vi "Track_overlay_test.vi"() -> ()   [LabVIEW 2018]
uses:
  Tracker.lvlib
panel:
  out "Color":u32(colorbox)=16711680
  out "Image Display 2":T1(plugin-control)
  out "Image Display":T1(plugin-control)
  out "error out":errorcluster
  in  "error in (no error)":errorcluster
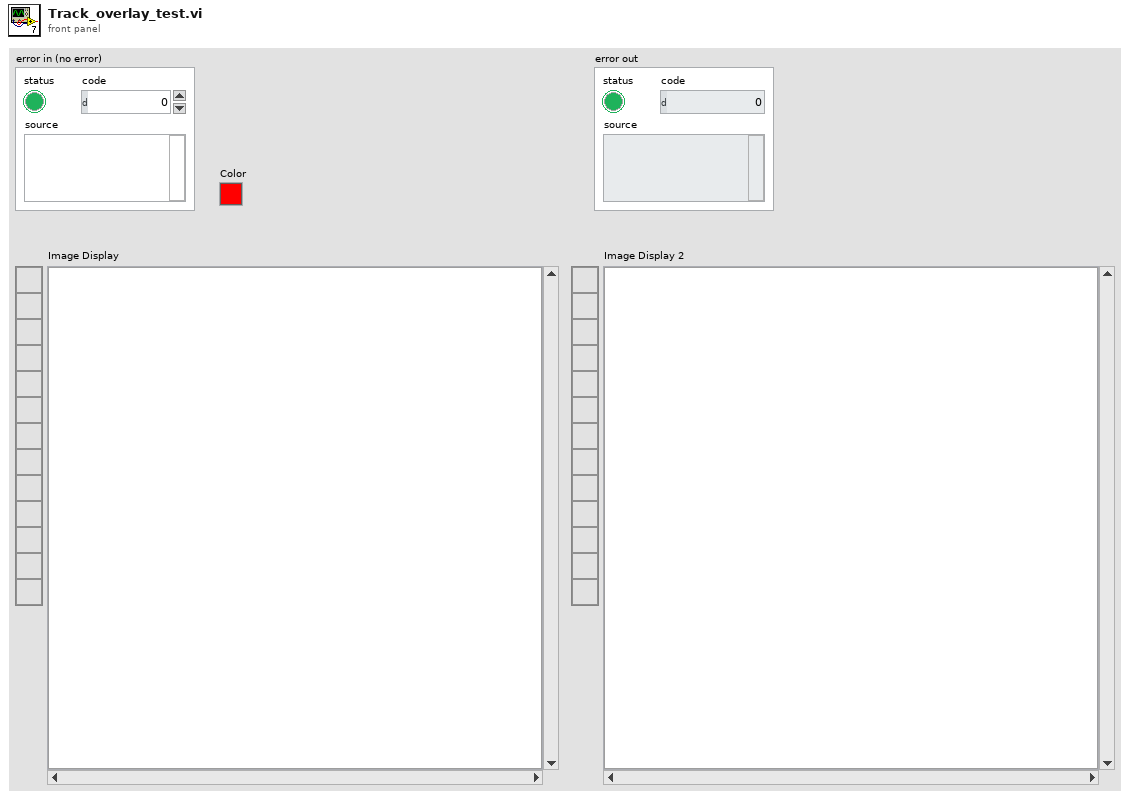
[diagram p1: front panel]
types:
  T1 = typedef "IMAQ Image.ctl" = refnum<image>
  T2 = cluster{"Left":i32, "Top":i32, "Right":i32, "Bottom":i32}
  T3 = typedef "Image Type" = u32
  T4 = cluster{"Numeric Control":dbl, "Numeric Control":dbl}[]
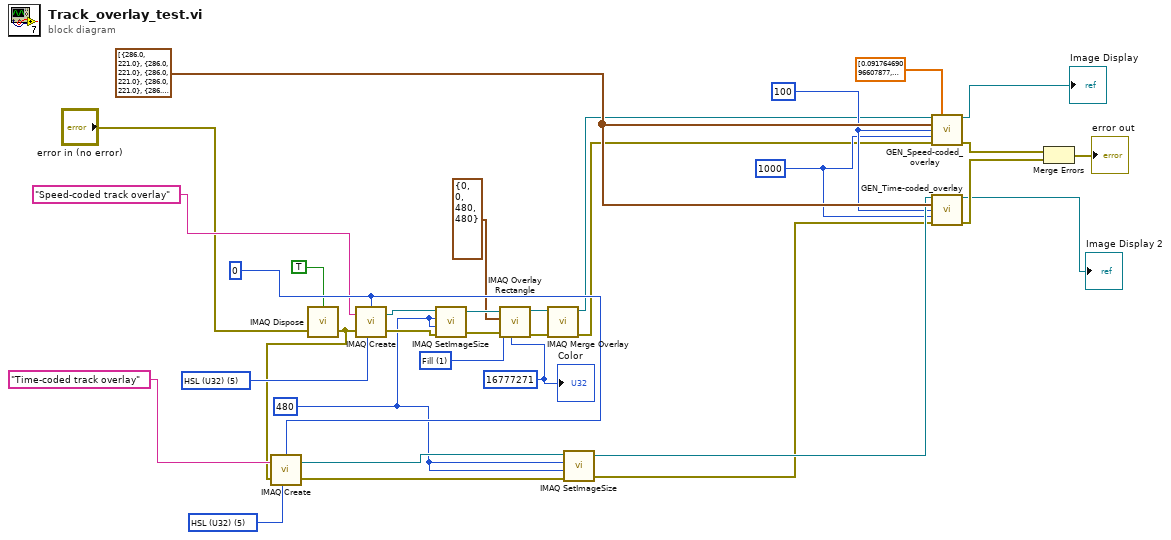
[diagram p0: block diagram]
diagram:
  w3 = u32 1 items=["Frame", "Fill", "Highlight"] ("Drawing Mode (Frame)")
  w5 = 16777271
  w21 = 0 ("Border Size")
  w23 = 1000 ("Samples full merge, every N")
  w24 = 100 ("Multiline grouping, samples")
  w18 = 480 ("X Resolution")
  w27 = T3 5 items=["Grayscale (U8)", "Grayscale (I16)", "Grayscale (SGL)", "Complex (CSG)", "RGB (U32)", "HSL (U32)", "RGB (U64)", "Grayscale (U16)"] ("Image Type")
  w20 = T3 5 items=["Grayscale (U8)", "Grayscale (I16)", "Grayscale (SGL)", "Complex (CSG)", "RGB (U32)", "HSL (U32)", "RGB (U64)", "Grayscale (U16)"] ("Image Type")
  w33 = T4 [{"Numeric Control"=286.0, "Numeric Control"=221.0}, {"Numeric Control"=286.0, "Numeric Control"=221.0}, {"Numeric Control"=286.0, "Numeric Control"=221.0}, {"Numeric Control"=286.0, "Numeric Control"=221.0}, {"Numeric Control"=286.0, "Numeric Control"=221.0}, {"Numeric Control"=286.0, "Numeric Control"=221.0}, {"Numeric Control"=286.0, "Numeric Control"=221.0}, {"Numeric Control"=286.0, "Numeric Control"=221.0}, {"Numeric Control"=286.0, "Numeric Control"=221.0}, {"Numeric Control"=285.0, "Numeric Control"=221.0}, {"Numeric Control"=285.0, "Numeric Control"=221.0}, {"Numeric Control"=285.0, "Numeric Control"=221.0}, {"Numeric Control"=285.0, "Numeric Control"=221.0}, {"Numeric Control"=285.0, "Numeric Control"=221.0}, {"Numeric Control"=285.0, "Numeric Control"=221.0}, {"Numeric Control"=285.0, "Numeric Control"=221.0}, {"Numeric Control"=285.0, "Numeric Control"=221.0}, {"Numeric Control"=285.0, "Numeric Control"=221.0}, {"Numeric Control"=285.0, "Numeric Control"=221.0}, {"Numeric Control"=285.0, "Numeric Control"=221.0}, {"Numeric Control"=285.0, "Numeric Control"=221.0}, {"Numeric Control"=285.0, "Numeric Control"=221.0}, {"Numeric Control"=285.0, "Numeric Control"=221.0}, {"Numeric Control"=285.0, "Numeric Control"=221.0}, {"Numeric Control"=285.0, "Numeric Control"=221.0}, {"Numeric Control"=285.0, "Numeric Control"=221.0}, {"Numeric Control"=286.0, "Numeric Control"=221.0}, {"Numeric Control"=286.0, "Numeric Control"=221.0}, {"Numeric Control"=285.0, "Numeric Control"=221.0}, {"Numeric Control"=286.0, "Numeric Control"=221.0}, {"Numeric Control"=286.0, "Numeric Control"=221.0}, {"Numeric Control"=286.0, "Numeric Control"=221.0}, {"Numeric Control"=285.0, "Numeric Control"=221.0}, {"Numeric Control"=286.0, "Numeric Control"=221.0}, {"Numeric Control"=286.0, "Numeric Control"=221.0}, {"Numeric Control"=286.0, "Numeric Control"=221.0}, {"Numeric Control"=286.0, "Numeric Control"=221.0}, {"Numeric Control"=286.0, "Numeric Control"=221.0}, {"Numeric Control"=286.0, "Numeric Control"=221.0}, {"Numeric Control"=286.0, "Numeric Control"=221.0}, {"Numeric Control"=286.0, "Numeric Control"=221.0}, {"Numeric Control"=286.0, "Numeric Control"=221.0}, {"Numeric Control"=286.0, "Numeric Control"=221.0}, {"Numeric Control"=286.0, "Numeric Control"=221.0}, {"Numeric Control"=286.0, "Numeric Control"=221.0}, {"Numeric Control"=286.0, "Numeric Control"=221.0}, {"Numeric Control"=285.0, "Numeric Control"=221.0}, {"Numeric Control"=285.0, "Numeric Control"=221.0}, {"Numeric Control"=285.0, "Numeric Control"=221.0}, {"Numeric Control"=285.0, "Numeric Control"=221.0}, {"Numeric Control"=285.0, "Numeric Control"=220.0}, {"Numeric Control"=285.0, "Numeric Control"=220.0}, {"Numeric Control"=285.0, "Numeric Control"=220.0}, {"Numeric Control"=285.0, "Numeric Control"=220.0}, {"Numeric Control"=285.0, "Numeric Control"=220.0}, {"Numeric Control"=285.0, "Numeric Control"=220.0}, {"Numeric Control"=285.0, "Numeric Control"=220.0}, {"Numeric Control"=285.0, "Numeric Control"=220.0}, {"Numeric Control"=285.0, "Numeric Control"=220.0}, {"Numeric Control"=285.0, "Numeric Control"=220.0}, {"Numeric Control"=285.0, "Numeric Control"=220.0}, {"Numeric Control"=285.0, "Numeric Control"=221.0}, {"Numeric Control"=285.0, "Numeric Control"=221.0}, {"Numeric Control"=285.0, "Numeric Control"=221.0}, {"Numeric Control"=285.0, "Numeric Control"=221.0}, {"Numeric Control"=285.0, "Numeric Control"=221.0}, {"Numeric Control"=285.0, "Numeric Control"=221.0}, {"Numeric Control"=285.0, "Numeric Control"=221.0}, {"Numeric Control"=285.0, "Numeric Control"=221.0}, {"Numeric Control"=285.0, "Numeric Control"=221.0}, {"Numeric Control"=285.0, "Numeric Control"=221.0}, {"Numeric Control"=286.0, "Numeric Control"=221.0}, {"Numeric Control"=286.0, "Numeric Control"=221.0}, {"Numeric Control"=286.0, "Numeric Control"=221.0}, {"Numeric Control"=286.0, "Numeric Control"=221.0}, {"Numeric Control"=286.0, "Numeric Control"=221.0}, {"Numeric Control"=286.0, "Numeric Control"=221.0}, {"Numeric Control"=286.0, "Numeric Control"=221.0}, {"Numeric Control"=286.0, "Numeric Control"=221.0}, {"Numeric Control"=286.0, "Numeric Control"=221.0}, {"Numeric Control"=286.0, "Numeric Control"=221.0}, {"Numeric Control"=286.0, "Numeric Control"=221.0}, {"Numeric Control"=286.0, "Numeric Control"=221.0}, {"Numeric Control"=286.0, "Numeric Control"=221.0}, {"Numeric Control"=286.0, "Numeric Control"=221.0}, {"Numeric Control"=286.0, "Numeric Control"=221.0}, {"Numeric Control"=286.0, "Numeric Control"=221.0}, {"Numeric Control"=286.0, "Numeric Control"=221.0}, {"Numeric Control"=286.0, "Numeric Control"=221.0}, {"Numeric Control"=286.0, "Numeric Control"=221.0}, {"Numeric Control"=286.0, "Numeric Control"=221.0}, {"Numeric Control"=286.0, "Numeric Control"=221.0}, {"Numeric Control"=286.0, "Numeric Control"=221.0}, {"Numeric Control"=286.0, "Numeric Control"=221.0}, {"Numeric Control"=286.0, "Numeric Control"=221.0}, {"Numeric Control"=286.0, "Numeric Control"=221.0}, {"Numeric Control"=286.0, "Numeric Control"=221.0}, {"Numeric Control"=286.0, "Numeric Control"=221.0}, {"Numeric Control"=286.0, "Numeric Control"=221.0}, {"Numeric Control"=286.0, "Numeric Control"=222.0}, {"Numeric Control"=286.0, "Numeric Control"=221.0}, {"Numeric Control"=286.0, "Numeric Control"=221.0}, {"Numeric Control"=286.0, "Numeric Control"=221.0}, {"Numeric Control"=286.0, "Numeric Control"=221.0}, {"Numeric Control"=286.0, "Numeric Control"=221.0}, {"Numeric Control"=286.0, "Numeric Control"=221.0}, {"Numeric Control"=286.0, "Numeric Control"=221.0}, {"Numeric Control"=286.0, "Numeric Control"=221.0}, {"Numeric Control"=286.0, "Numeric Control"=221.0}, {"Numeric Control"=286.0, "Numeric Control"=221.0}, {"Numeric Control"=286.0, "Numeric Control"=221.0}, {"Numeric Control"=286.0, "Numeric Control"=221.0}, {"Numeric Control"=286.0, "Numeric Control"=221.0}, {"Numeric Control"=286.0, "Numeric Control"=221.0}, {"Numeric Control"=286.0, "Numeric Control"=221.0}, {"Numeric Control"=286.0, "Numeric Control"=221.0}, {"Numeric Control"=286.0, "Numeric Control"=221.0}, {"Numeric Control"=286.0, "Numeric Control"=221.0}, {"Numeric Control"=286.0, "Numeric Control"=221.0}, {"Numeric Control"=286.0, "Numeric Control"=221.0}, {"Numeric Control"=286.0, "Numeric Control"=221.0}, {"Numeric Control"=286.0, "Numeric Control"=221.0}, {"Numeric Control"=286.0, "Numeric Control"=221.0}, {"Numeric Control"=286.0, "Numeric Control"=221.0}, {"Numeric Control"=286.0, "Numeric Control"=220.0}, {"Numeric Control"=286.0, "Numeric Control"=220.0}, {"Numeric Control"=286.0, "Numeric Control"=220.0}, {"Numeric Control"=286.0, "Numeric Control"=220.0}, {"Numeric Control"=286.0, "Numeric Control"=221.0}, {"Numeric Control"=286.0, "Numeric Control"=221.0}, {"Numeric Control"=286.0, "Numeric Control"=221.0}, {"Numeric Control"=286.0, "Numeric Control"=221.0}, {"Numeric Control"=286.0, "Numeric Control"=222.0}, {"Numeric Control"=285.0, "Numeric Control"=222.0}, {"Numeric Control"=285.0, "Numeric Control"=223.0}, {"Numeric Control"=285.0, "Numeric Control"=223.0}, {"Numeric Control"=285.0, "Numeric Control"=224.0}, {"Numeric Control"=285.0, "Numeric Control"=225.0}, {"Numeric Control"=284.0, "Numeric Control"=225.0}, {"Numeric Control"=284.0, "Numeric Control"=226.0}, {"Numeric Control"=283.0, "Numeric Control"=227.0}, {"Numeric Control"=282.0, "Numeric Control"=228.0}, {"Numeric Control"=281.0, "Numeric Control"=229.0}, {"Numeric Control"=280.0, "Numeric Control"=229.0}, {"Numeric Control"=278.0, "Numeric Control"=230.0}, {"Numeric Control"=277.0, "Numeric Control"=231.0}, {"Numeric Control"=275.0, "Numeric Control"=232.0}, {"Numeric Control"=274.0, "Numeric Control"=233.0}, {"Numeric Control"=272.0, "Numeric Control"=234.0}, {"Numeric Control"=270.0, "Numeric Control"=235.0}, {"Numeric Control"=269.0, "Numeric Control"=235.0}, {"Numeric Control"=267.0, "Numeric Control"=236.0}, {"Numeric Control"=265.0, "Numeric Control"=236.0}, {"Numeric Control"=263.0, "Numeric Control"=236.0}, {"Numeric Control"=260.0, "Numeric Control"=235.0}, {"Numeric Control"=258.0, "Numeric Control"=235.0}, {"Numeric Control"=256.0, "Numeric Control"=233.0}, {"Numeric Control"=253.0, "Numeric Control"=232.0}, {"Numeric Control"=251.0, "Numeric Control"=231.0}, {"Numeric Control"=248.0, "Numeric Control"=228.0}, {"Numeric Control"=246.0, "Numeric Control"=226.0}, {"Numeric Control"=244.0, "Numeric Control"=223.0}, {"Numeric Control"=242.0, "Numeric Control"=220.0}, {"Numeric Control"=240.0, "Numeric Control"=217.0}, {"Numeric Control"=240.0, "Numeric Control"=214.0}, {"Numeric Control"=239.0, "Numeric Control"=210.0}, {"Numeric Control"=240.0, "Numeric Control"=207.0}, {"Numeric Control"=241.0, "Numeric Control"=203.0}, {"Numeric Control"=242.0, "Numeric Control"=200.0}, {"Numeric Control"=245.0, "Numeric Control"=196.0}, {"Numeric Control"=248.0, "Numeric Control"=194.0}, {"Numeric Control"=252.0, "Numeric Control"=191.0}, {"Numeric Control"=257.0, "Numeric Control"=189.0}, {"Numeric Control"=262.0, "Numeric Control"=188.0}, {"Numeric Control"=269.0, "Numeric Control"=187.0}, {"Numeric Control"=276.0, "Numeric Control"=187.0}, {"Numeric Control"=283.0, "Numeric Control"=188.0}, {"Numeric Control"=291.0, "Numeric Control"=190.0}, {"Numeric Control"=299.0, "Numeric Control"=193.0}, {"Numeric Control"=306.0, "Numeric Control"=198.0}, {"Numeric Control"=314.0, "Numeric Control"=203.0}, {"Numeric Control"=321.0, "Numeric Control"=210.0}, {"Numeric Control"=327.0, "Numeric Control"=217.0}, {"Numeric Control"=332.0, "Numeric Control"=226.0}, {"Numeric Control"=336.0, "Numeric Control"=235.0}, {"Numeric Control"=339.0, "Numeric Control"=244.0}, {"Numeric Control"=341.0, "Numeric Control"=253.0}, {"Numeric Control"=341.0, "Numeric Control"=262.0}, {"Numeric Control"=340.0, "Numeric Control"=271.0}, {"Numeric Control"=338.0, "Numeric Control"=280.0}, {"Numeric Control"=334.0, "Numeric Control"=288.0}, {"Numeric Control"=329.0, "Numeric Control"=295.0}, {"Numeric Control"=323.0, "Numeric Control"=300.0}, {"Numeric Control"=316.0, "Numeric Control"=306.0}, {"Numeric Control"=307.0, "Numeric Control"=309.0}, {"Numeric Control"=298.0, "Numeric Control"=312.0}, {"Numeric Control"=288.0, "Numeric Control"=313.0}, {"Numeric Control"=277.0, "Numeric Control"=313.0}, {"Numeric Control"=267.0, "Numeric Control"=311.0}, {"Numeric Control"=257.0, "Numeric Control"=309.0}, {"Numeric Control"=246.0, "Numeric Control"=305.0}, {"Numeric Control"=236.0, "Numeric Control"=300.0}, {"Numeric Control"=226.0, "Numeric Control"=295.0}, {"Numeric Control"=216.0, "Numeric Control"=289.0}, {"Numeric Control"=207.0, "Numeric Control"=282.0}, {"Numeric Control"=199.0, "Numeric Control"=275.0}, {"Numeric Control"=191.0, "Numeric Control"=267.0}, {"Numeric Control"=183.0, "Numeric Control"=259.0}, {"Numeric Control"=177.0, "Numeric Control"=251.0}, {"Numeric Control"=172.0, "Numeric Control"=243.0}, {"Numeric Control"=169.0, "Numeric Control"=235.0}, {"Numeric Control"=167.0, "Numeric Control"=226.0}, {"Numeric Control"=166.0, "Numeric Control"=218.0}, {"Numeric Control"=167.0, "Numeric Control"=210.0}, {"Numeric Control"=170.0, "Numeric Control"=202.0}, {"Numeric Control"=174.0, "Numeric Control"=195.0}, {"Numeric Control"=180.0, "Numeric Control"=189.0}, {"Numeric Control"=187.0, "Numeric Control"=184.0}, {"Numeric Control"=196.0, "Numeric Control"=180.0}, {"Numeric Control"=206.0, "Numeric Control"=177.0}, {"Numeric Control"=217.0, "Numeric Control"=176.0}, {"Numeric Control"=228.0, "Numeric Control"=176.0}, {"Numeric Control"=239.0, "Numeric Control"=177.0}, {"Numeric Control"=250.0, "Numeric Control"=179.0}, {"Numeric Control"=261.0, "Numeric Control"=183.0}, {"Numeric Control"=271.0, "Numeric Control"=188.0}, {"Numeric Control"=280.0, "Numeric Control"=194.0}, {"Numeric Control"=288.0, "Numeric Control"=202.0}, {"Numeric Control"=295.0, "Numeric Control"=210.0}, {"Numeric Control"=301.0, "Numeric Control"=219.0}, {"Numeric Control"=304.0, "Numeric Control"=228.0}, {"Numeric Control"=306.0, "Numeric Control"=237.0}, {"Numeric Control"=307.0, "Numeric Control"=246.0}, {"Numeric Control"=307.0, "Numeric Control"=254.0}, {"Numeric Control"=304.0, "Numeric Control"=262.0}, {"Numeric Control"=300.0, "Numeric Control"=268.0}, {"Numeric Control"=295.0, "Numeric Control"=273.0}, {"Numeric Control"=289.0, "Numeric Control"=277.0}, {"Numeric Control"=282.0, "Numeric Control"=280.0}, {"Numeric Control"=273.0, "Numeric Control"=281.0}, {"Numeric Control"=264.0, "Numeric Control"=281.0}, {"Numeric Control"=255.0, "Numeric Control"=279.0}, {"Numeric Control"=245.0, "Numeric Control"=277.0}, {"Numeric Control"=236.0, "Numeric Control"=273.0}, {"Numeric Control"=226.0, "Numeric Control"=269.0}, {"Numeric Control"=216.0, "Numeric Control"=264.0}, {"Numeric Control"=206.0, "Numeric Control"=258.0}, {"Numeric Control"=197.0, "Numeric Control"=251.0}, {"Numeric Control"=188.0, "Numeric Control"=245.0}, {"Numeric Control"=181.0, "Numeric Control"=238.0}, {"Numeric Control"=174.0, "Numeric Control"=231.0}, {"Numeric Control"=168.0, "Numeric Control"=224.0}, {"Numeric Control"=163.0, "Numeric Control"=216.0}, {"Numeric Control"=160.0, "Numeric Control"=209.0}, {"Numeric Control"=157.0, "Numeric Control"=201.0}, {"Numeric Control"=156.0, "Numeric Control"=194.0}, {"Numeric Control"=157.0, "Numeric Control"=187.0}, {"Numeric Control"=159.0, "Numeric Control"=180.0}, {"Numeric Control"=163.0, "Numeric Control"=173.0}, {"Numeric Control"=168.0, "Numeric Control"=167.0}, {"Numeric Control"=175.0, "Numeric Control"=162.0}, {"Numeric Control"=182.0, "Numeric Control"=158.0}, {"Numeric Control"=190.0, "Numeric Control"=155.0}, {"Numeric Control"=199.0, "Numeric Control"=153.0}, {"Numeric Control"=209.0, "Numeric Control"=152.0}, {"Numeric Control"=218.0, "Numeric Control"=152.0}, {"Numeric Control"=228.0, "Numeric Control"=154.0}, {"Numeric Control"=237.0, "Numeric Control"=157.0}, {"Numeric Control"=246.0, "Numeric Control"=161.0}, {"Numeric Control"=254.0, "Numeric Control"=167.0}, {"Numeric Control"=261.0, "Numeric Control"=173.0}, {"Numeric Control"=267.0, "Numeric Control"=179.0}, {"Numeric Control"=272.0, "Numeric Control"=186.0}, {"Numeric Control"=275.0, "Numeric Control"=193.0}, {"Numeric Control"=277.0, "Numeric Control"=200.0}, {"Numeric Control"=277.0, "Numeric Control"=206.0}, {"Numeric Control"=276.0, "Numeric Control"=212.0}, {"Numeric Control"=274.0, "Numeric Control"=218.0}, {"Numeric Control"=271.0, "Numeric Control"=223.0}, {"Numeric Control"=267.0, "Numeric Control"=227.0}, {"Numeric Control"=262.0, "Numeric Control"=231.0}, {"Numeric Control"=256.0, "Numeric Control"=235.0}, {"Numeric Control"=251.0, "Numeric Control"=237.0}, {"Numeric Control"=244.0, "Numeric Control"=240.0}, {"Numeric Control"=237.0, "Numeric Control"=241.0}, {"Numeric Control"=230.0, "Numeric Control"=242.0}, {"Numeric Control"=223.0, "Numeric Control"=243.0}, {"Numeric Control"=215.0, "Numeric Control"=243.0}, {"Numeric Control"=209.0, "Numeric Control"=243.0}, {"Numeric Control"=202.0, "Numeric Control"=243.0}, {"Numeric Control"=195.0, "Numeric Control"=242.0}, {"Numeric Control"=190.0, "Numeric Control"=241.0}, {"Numeric Control"=184.0, "Numeric Control"=240.0}, {"Numeric Control"=179.0, "Numeric Control"=239.0}, {"Numeric Control"=174.0, "Numeric Control"=237.0}, {"Numeric Control"=170.0, "Numeric Control"=235.0}, {"Numeric Control"=167.0, "Numeric Control"=234.0}, {"Numeric Control"=164.0, "Numeric Control"=232.0}, {"Numeric Control"=162.0, "Numeric Control"=231.0}, {"Numeric Control"=160.0, "Numeric Control"=229.0}, {"Numeric Control"=159.0, "Numeric Control"=228.0}, {"Numeric Control"=159.0, "Numeric Control"=227.0}, {"Numeric Control"=159.0, "Numeric Control"=226.0}, {"Numeric Control"=159.0, "Numeric Control"=225.0}, {"Numeric Control"=159.0, "Numeric Control"=225.0}, {"Numeric Control"=159.0, "Numeric Control"=224.0}, {"Numeric Control"=160.0, "Numeric Control"=224.0}, {"Numeric Control"=161.0, "Numeric Control"=224.0}, {"Numeric Control"=161.0, "Numeric Control"=224.0}, {"Numeric Control"=162.0, "Numeric Control"=224.0}, {"Numeric Control"=163.0, "Numeric Control"=224.0}, {"Numeric Control"=164.0, "Numeric Control"=224.0}, {"Numeric Control"=165.0, "Numeric Control"=224.0}, {"Numeric Control"=165.0, "Numeric Control"=223.0}, {"Numeric Control"=166.0, "Numeric Control"=223.0}, {"Numeric Control"=166.0, "Numeric Control"=223.0}, {"Numeric Control"=167.0, "Numeric Control"=223.0}, {"Numeric Control"=167.0, "Numeric Control"=223.0}, {"Numeric Control"=167.0, "Numeric Control"=223.0}, {"Numeric Control"=167.0, "Numeric Control"=223.0}, {"Numeric Control"=167.0, "Numeric Control"=223.0}, {"Numeric Control"=168.0, "Numeric Control"=223.0}, {"Numeric Control"=168.0, "Numeric Control"=223.0}, {"Numeric Control"=168.0, "Numeric Control"=223.0}, {"Numeric Control"=168.0, "Numeric Control"=223.0}, {"Numeric Control"=168.0, "Numeric Control"=223.0}, {"Numeric Control"=168.0, "Numeric Control"=223.0}, {"Numeric Control"=168.0, "Numeric Control"=223.0}, {"Numeric Control"=168.0, "Numeric Control"=223.0}, {"Numeric Control"=168.0, "Numeric Control"=223.0}, {"Numeric Control"=168.0, "Numeric Control"=223.0}, {"Numeric Control"=168.0, "Numeric Control"=223.0}, {"Numeric Control"=168.0, "Numeric Control"=223.0}, {"Numeric Control"=168.0, "Numeric Control"=223.0}, {"Numeric Control"=168.0, "Numeric Control"=223.0}, {"Numeric Control"=168.0, "Numeric Control"=223.0}, {"Numeric Control"=168.0, "Numeric Control"=223.0}, {"Numeric Control"=168.0, "Numeric Control"=223.0}, {"Numeric Control"=168.0, "Numeric Control"=222.0}, {"Numeric Control"=168.0, "Numeric Control"=222.0}, {"Numeric Control"=168.0, "Numeric Control"=222.0}, {"Numeric Control"=168.0, "Numeric Control"=222.0}, {"Numeric Control"=168.0, "Numeric Control"=222.0}, {"Numeric Control"=168.0, "Numeric Control"=222.0}, {"Numeric Control"=168.0, "Numeric Control"=222.0}, {"Numeric Control"=168.0, "Numeric Control"=222.0}, {"Numeric Control"=168.0, "Numeric Control"=222.0}, {"Numeric Control"=168.0, "Numeric Control"=222.0}, {"Numeric Control"=168.0, "Numeric Control"=222.0}, {"Numeric Control"=168.0, "Numeric Control"=222.0}, {"Numeric Control"=168.0, "Numeric Control"=222.0}, {"Numeric Control"=168.0, "Numeric Control"=222.0}, {"Numeric Control"=168.0, "Numeric Control"=222.0}, {"Numeric Control"=168.0, "Numeric Control"=222.0}, {"Numeric Control"=168.0, "Numeric Control"=223.0}, {"Numeric Control"=168.0, "Numeric Control"=223.0}, {"Numeric Control"=168.0, "Numeric Control"=223.0}, {"Numeric Control"=168.0, "Numeric Control"=223.0}, {"Numeric Control"=168.0, "Numeric Control"=223.0}, {"Numeric Control"=168.0, "Numeric Control"=223.0}, {"Numeric Control"=168.0, "Numeric Control"=223.0}, {"Numeric Control"=168.0, "Numeric Control"=223.0}, {"Numeric Control"=168.0, "Numeric Control"=223.0}, {"Numeric Control"=168.0, "Numeric Control"=223.0}, {"Numeric Control"=168.0, "Numeric Control"=223.0}, {"Numeric Control"=168.0, "Numeric Control"=223.0}, {"Numeric Control"=168.0, "Numeric Control"=223.0}, {"Numeric Control"=168.0, "Numeric Control"=223.0}, {"Numeric Control"=168.0, "Numeric Control"=223.0}, {"Numeric Control"=168.0, "Numeric Control"=223.0}, {"Numeric Control"=168.0, "Numeric Control"=223.0}, {"Numeric Control"=168.0, "Numeric Control"=223.0}, {"Numeric Control"=168.0, "Numeric Control"=223.0}, {"Numeric Control"=168.0, "Numeric Control"=223.0}, {"Numeric Control"=168.0, "Numeric Control"=223.0}, {"Numeric Control"=168.0, "Numeric Control"=223.0}, {"Numeric Control"=168.0, "Numeric Control"=223.0}, {"Numeric Control"=168.0, "Numeric Control"=223.0}, {"Numeric Control"=168.0, "Numeric Control"=223.0}, {"Numeric Control"=168.0, "Numeric Control"=223.0}, {"Numeric Control"=168.0, "Numeric Control"=223.0}, {"Numeric Control"=168.0, "Numeric Control"=223.0}, {"Numeric Control"=168.0, "Numeric Control"=223.0}, {"Numeric Control"=168.0, "Numeric Control"=223.0}, {"Numeric Control"=168.0, "Numeric Control"=223.0}, {"Numeric Control"=168.0, "Numeric Control"=223.0}, {"Numeric Control"=168.0, "Numeric Control"=223.0}, {"Numeric Control"=168.0, "Numeric Control"=223.0}, {"Numeric Control"=168.0, "Numeric Control"=223.0}, {"Numeric Control"=168.0, "Numeric Control"=224.0}, {"Numeric Control"=168.0, "Numeric Control"=223.0}, {"Numeric Control"=168.0, "Numeric Control"=224.0}, {"Numeric Control"=168.0, "Numeric Control"=224.0}, {"Numeric Control"=168.0, "Numeric Control"=223.0}, {"Numeric Control"=168.0, "Numeric Control"=224.0}, {"Numeric Control"=168.0, "Numeric Control"=223.0}, {"Numeric Control"=168.0, "Numeric Control"=224.0}, {"Numeric Control"=168.0, "Numeric Control"=223.0}, {"Numeric Control"=168.0, "Numeric Control"=223.0}, {"Numeric Control"=168.0, "Numeric Control"=223.0}, {"Numeric Control"=168.0, "Numeric Control"=223.0}, {"Numeric Control"=168.0, "Numeric Control"=223.0}, {"Numeric Control"=168.0, "Numeric Control"=223.0}, {"Numeric Control"=168.0, "Numeric Control"=223.0}, {"Numeric Control"=168.0, "Numeric Control"=222.0}, {"Numeric Control"=168.0, "Numeric Control"=223.0}, {"Numeric Control"=168.0, "Numeric Control"=222.0}, {"Numeric Control"=168.0, "Numeric Control"=222.0}, {"Numeric Control"=168.0, "Numeric Control"=222.0}, {"Numeric Control"=168.0, "Numeric Control"=222.0}, {"Numeric Control"=168.0, "Numeric Control"=223.0}, {"Numeric Control"=168.0, "Numeric Control"=222.0}, {"Numeric Control"=168.0, "Numeric Control"=222.0}, {"Numeric Control"=168.0, "Numeric Control"=222.0}, {"Numeric Control"=168.0, "Numeric Control"=222.0}, {"Numeric Control"=168.0, "Numeric Control"=222.0}, {"Numeric Control"=168.0, "Numeric Control"=222.0}, {"Numeric Control"=168.0, "Numeric Control"=222.0}, {"Numeric Control"=168.0, "Numeric Control"=222.0}, {"Numeric Control"=168.0, "Numeric Control"=222.0}, {"Numeric Control"=168.0, "Numeric Control"=222.0}, {"Numeric Control"=168.0, "Numeric Control"=222.0}, {"Numeric Control"=168.0, "Numeric Control"=222.0}, {"Numeric Control"=168.0, "Numeric Control"=222.0}, {"Numeric Control"=168.0, "Numeric Control"=222.0}, {"Numeric Control"=168.0, "Numeric Control"=223.0}, {"Numeric Control"=168.0, "Numeric Control"=223.0}, {"Numeric Control"=168.0, "Numeric Control"=223.0}, {"Numeric Control"=168.0, "Numeric Control"=223.0}, {"Numeric Control"=168.0, "Numeric Control"=222.0}, {"Numeric Control"=168.0, "Numeric Control"=222.0}, {"Numeric Control"=168.0, "Numeric Control"=222.0}, {"Numeric Control"=168.0, "Numeric Control"=222.0}, {"Numeric Control"=168.0, "Numeric Control"=222.0}, {"Numeric Control"=168.0, "Numeric Control"=222.0}, {"Numeric Control"=168.0, "Numeric Control"=222.0}, {"Numeric Control"=168.0, "Numeric Control"=222.0}, {"Numeric Control"=168.0, "Numeric Control"=222.0}, {"Numeric Control"=168.0, "Numeric Control"=222.0}, {"Numeric Control"=168.0, "Numeric Control"=222.0}, {"Numeric Control"=168.0, "Numeric Control"=222.0}, {"Numeric Control"=168.0, "Numeric Control"=222.0}, {"Numeric Control"=168.0, "Numeric Control"=222.0}, {"Numeric Control"=168.0, "Numeric Control"=222.0}, {"Numeric Control"=168.0, "Numeric Control"=222.0}, {"Numeric Control"=168.0, "Numeric Control"=222.0}, {"Numeric Control"=167.0, "Numeric Control"=222.0}, {"Numeric Control"=167.0, "Numeric Control"=222.0}] ("Full track array")
  n1 = call "IMAQ Dispose"("All Images? (No)"=TRUE, "error in (no error)"="error in (no error)") -> ("error out"=w10:errorcluster)  [unwired: 4 in]
  n2 = call "IMAQ Create"("Border Size"=w21, "Image Name"="Time-coded track overlay", "Image Type"=w27, "error in (no error)"=w10) -> ("New Image"=w28:T1, "error out"=w26:errorcluster)  [unwired: 1 in]
  n3 = call "IMAQ Create"("Border Size"=w21, "Image Name"="Speed-coded track overlay", "Image Type"=w20, "error in (no error)"=w10) -> ("New Image"=w17:T1, "error out"=w19:errorcluster)  [unwired: 1 in]
  n4 = call "IMAQ SetImageSize"("error in (no error)"=w19, "Y Resolution"=w18, "X Resolution"=w18, "Image"=w17) -> ("error out"=w6:errorcluster, "Image Out"=w7:T1)  [unwired: 1 in]
  n5 = call "IMAQ Overlay Rectangle"("Color"=w5, "error in (no error)"=w6, "Drawing Mode (Frame)"=w3, "Rectangle"=T2 {"Left"=0, "Top"=0, "Right"=480, "Bottom"=480}, "Image"=w7) -> ("error out"=w9:errorcluster, "Image Out"=w8:T1)  [unwired: 5 in]
  n6 = call "IMAQ Merge Overlay"("error in (no error)"=w9, "Image Src"=w8) -> ("error out"=w1:errorcluster, "Image Dst Out"=w2:T1)  [unwired: 8 in]
  n7 = call "IMAQ SetImageSize"("error in (no error)"=w26, "Y Resolution"=w18, "X Resolution"=w18, "Image"=w28) -> ("error out"=w16:errorcluster, "Image Out"=w25:T1)  [unwired: 1 in]
  n8 = call "GEN_Speed-coded_overlay.vi"("Speed-coded overlay refnum in"=w2, "Speed array in"=dbl[] [0.09176469096607877, 1.2846150032484263, 8.349236020736805, 33.392883301810905, 91.81495742012963, 183.58493789522015, 275.2732272720206, 314.39936590454107, 274.7793083320438, 182.73935449749104, 90.81877822233525, 32.42325838923357, 7.594873795777121, 1.6373335941766733, 1.6448034316578672, 1.5990520129165509, 1.5187563411167864, 1.4388992074402887, 1.3589503869536108, 1.2784373333723154, 1.1969629122629173, 1.114237943833408, 1.030169209133307, 0.9448620817615184, 0.8575084951181364, 0.7630797575626084, 0.6507923418056639, 0.5146872743052909, 0.3862352766345853, 0.3886014274744571, 0.5891625018605106, 0.8463732830818489, 0.9960028508763307, 0.9325090580171058, 0.6957534024080986, 0.45001488790986693, 0.34032008112166257, 0.3812990782204667, 0.5537131323421934, 0.865865915170671, 1.286277992827452, 1.798054337947497, 2.428031137080297, 3.102990033657568, 3.503993901257993, 3.2060031439128607, 2.0415765508604733, 0.34182835577198045, 1.6084346271654337, 3.1006737657776196, 4.064092520852645, 4.53851753921977, 4.666811170752466, 4.5948491013738355, 4.450398612877405, 4.300223848282913, 4.042992390861234, 3.4471653318618283, 2.440679319655425, 1.3277523950547863, 0.6495349787840039, 0.5829995956565679, 0.5953122795454817, 0.6115549624433261, 0.8779443599053179, 1.4946094189000227, 2.150348411005169, 2.4957722216325413, 2.369920442494217, 1.87847244827897, 1.2997209238343688, 0.8740226117251237, 0.6520408433571285, 0.5582606331216869, 0.5860573040599781, 0.8475950169367676, 1.4091250249041973, 2.144041556997857, 2.8074323139653887, 3.233099477488566, 3.4284862269322662, 3.459571809868631, 3.2567797928558573, 2.596729319738284, 1.3529894324253406, 0.3542805166049301, 1.6547545767172833, 2.221716188263466, 1.8694222497435844, 1.0087332170521168, 0.37146762881147877, 0.28800953436145904, 0.32655536790506273, 0.5977757306895702, 0.5916890680798474, 0.25648698288056004, 0.3957434169182052, 0.7386685165064744, 0.87593492169617, 0.922600368708977, 1.0823488101271905, 1.4883118214432802, 2.0929085753624017, 2.720818752769156, 3.10134023851595, 2.910585212219752, 1.9831708565974735, 0.5605206340752765, 0.7999445698101727, 1.4885280456987637, 1.4022805126450781, 0.9179194914547764, 0.5917545820234245, 0.6084487491200075, 0.9204119056165027, 1.2550123481556292, 1.309346970956699, 1.0670855926394323, 0.7242456886819126, 0.4964329359397094, 0.45361470741230747, 0.6087716383977346, 1.0945875260403573, 1.8456605562051462, 2.585832472259349, 3.0258525732684625, 3.0493273425455456, 2.7329445871799187, 2.2402079123440473, 1.8373271125740274, 1.813406813791609, 1.9216073701270235, 1.7147961557742306, 1.5293146510938838, 2.4659842601758926, 4.048892370015907, 5.664635283867369, 7.324662541725609, 9.273032541566852, 11.604387478860795, 14.195284281525444, 16.80671692912072, 19.23624163281531, 21.48932522080623, 23.820624692693084, 26.5771814304915, 29.925878252272405, 33.70109324836196, 37.55174011163381, 41.205825684919965, 44.574935162180836, 47.673218485282696, 50.472808535424704, 52.83005013965195, 54.58067988321516, 55.72705239685157, 56.506885687451664, 57.28060141265327, 58.38308856646977, 60.096838440934725, 62.73500501880198, 66.63609905240956, 71.93425237896223, 78.28707121499689, 84.88795731370674, 90.82949771210156, 95.51454257052096, 98.74468602600122, 100.5571466699339, 101.23432898606588, 101.45414174030999, 102.06708057533656, 103.51881655964043, 105.67589648357827, 108.410547278887, 112.26540606935473, 118.38165810283954, 127.74978425270065, 140.53737532886242, 155.99103094404646, 172.794333407837, 189.58804428890517, 205.42893796399522, 220.01621259628607, 233.5912927848129, 246.51072106441188, 258.72175174964235, 269.57967580501185, 278.15151993858757, 283.6545022949217, 285.6837409501936, 284.2994887925627, 280.180075010341, 274.6090371250267, 268.8875385125523, 263.5677068495883, 258.5664828574853, 254.2558065474191, 252.1152594791501, 253.91823470143805, 260.3522282601302, 270.51010983892706, 282.3670436492194, 293.72158292264334, 303.26565735159176, 311.1179407714437, 318.2326564168819, 325.2070294660488, 331.66157404895296, 336.6247398017535, 339.2668401141931, 339.1288743759566, 335.7404810998, 328.37868850088944, 316.6034786911799, 301.1261585270232, 283.9629120036343, 267.55255324676955, 253.65575690361663, 243.04346841566394, 236.09396774900165, 233.52476477975085, 236.4237966382317, 245.4391625709732, 259.8513701370278, 277.39468522355116, 294.99667199167726, 309.99338351663846, 321.0935023648253, 328.3766862249856, 332.39163593805034, 333.40639318548847, 331.5579177526036, 327.2441339558032, 320.7777569686328, 311.81879400054174, 299.83482240115734, 285.1347269408053, 268.9480824836026, 252.64479625115797, 237.43476713793254, 224.68793398068829, 215.9873325856869, 212.87769315607187, 216.57971436914204, 227.18401656772912, 242.81081267626791, 260.2940054307721, 277.0478917177601, 292.15249845645627, 305.773314144393, 317.73897043233944, 326.72791747329916, 330.82109164137205, 328.8456387774859, 321.1959727623882, 309.4155947174553, 295.11885876288784, 279.3497332045946, 262.7588064045968, 246.17550978197102, 231.09493154832404, 219.70375277063647, 214.02755417959133, 214.53700621970867, 219.76361333923032, 227.58505102312986, 236.6520818882523, 246.5052662921764, 256.6841993450196, 266.1422771857608, 273.69106774672446, 278.80597243825315, 281.67423764535675, 282.4342281448096, 280.63545599709204, 275.51928908439504, 266.63221564689496, 254.1786915357386, 239.05328744892236, 222.63657496859352, 206.46878384935673, 192.15298681311222, 181.51251232022943, 176.19541513540096, 176.43559465091107, 180.52805746362284, 186.1650149614073, 192.06952416969278, 198.10566540728342, 204.19758164329542, 209.5572669328017, 212.95448932126988, 213.49765880633606, 211.09024302626227, 206.2627344780912, 199.64615883811337, 191.5509627683016, 181.91778134845688, 170.55320809915423, 157.4118577688244, 142.76760492266226, 127.18994984590914, 111.29950885694116, 95.47626949036193, 79.83663715122833, 64.55853687037597, 50.24141195821128, 37.94361783104842, 28.796967504093182, 23.242306655881574, 20.448254334919792, 19.16872064799645, 19.061566206312833, 20.347594418273545, 22.552631898624156, 24.421979925030453, 24.915194707818017, 23.84665411958587, 21.726201125331926, 19.178559360947155, 16.52859267330818, 13.826292170225116, 11.159021163566914, 8.843090366735424, 7.185752447274747, 6.13722391173328, 5.428553308654203, 4.783164505031111, 3.8887963499994953, 2.6309438849920546, 1.3110874807309456, 0.7973682779770128, 1.3425861966020862, 1.76516900864048, 1.8462742466419781, 1.6089456782567584, 1.1788457943610136, 0.8767548851547662, 1.368159367916189, 2.383032470364076, 3.338266968632267, 3.826744623607673, 3.720159735879307, 3.222698566181885, 2.666652936645811, 2.2781379888517037, 2.121726062404242, 2.151985374123686, 2.2099471652139537, 2.087920786299889, 1.6928239247540018, 1.0974947952600012, 0.47036707186802573, 0.42535620576229455, 0.9281601505623389, 1.3334185093234243, 1.6187057642870966, 1.928048134428133, 2.43233496128316, 3.0509962708816682, 3.462905867950034, 3.3750985057318763, 2.7035397481183514, 1.6602854330675267, 0.6946079919894947, 0.276299265494592, 0.3593532899976697, 0.7535166417200035, 1.284313661992559, 1.6683153075886554, 1.762137397267336, 1.5684159369304387, 1.1882642132438215, 0.758985524712651, 0.40035584990136003, 0.15586608374571517, 0.12525798803926816, 0.4726814841559691, 0.9699921217017313, 1.3844624252519893, 1.43306525506847, 1.0603218051679881, 0.5430693488176827, 0.3489234957402871, 0.37732709986803253, 0.3654632307270141, 0.43765786710961396, 0.5636943479981001, 0.7229432171693917, 0.9627082832344159, 1.3683551957091058, 2.0276116190291216, 2.8612126684064614, 3.5552247130460124, 3.7633942659406547, 3.375366508540654, 2.561029660978697, 1.5918352366896709, 0.7237861610099406, 0.587256355058316, 1.2071204111853184, 1.9615448239619302, 2.7903847627553895, 3.4542249488444616, 3.6290433563170215, 3.2960721007484453, 2.840449153405214, 2.65004468151371, 2.6899463918271356, 2.61982220407554, 2.2355798526678057, 1.6664092940350967, 1.1700361466292044, 0.9284299914601487, 1.014761142239424, 1.2609488190762332, 1.5090309797531238, 1.7434631375666432, 1.870430024361779, 1.8031874028996357, 1.6078525887606492, 1.3974470113541084, 1.216949031394948, 1.0422485318497539, 0.7860916542843084, 0.3858749266632915, 0.6159305710366219, 1.4917637127658785, 2.3102966200761026, 2.751936935305338, 2.673460089524923, 2.1175834029689495, 1.2354010918121792, 0.37501543742628846, 0.9356820384127866, 1.675127870274153, 2.161861683705643, 2.4278624458814133, 2.5514272874636403, 2.591700605963674, 2.5767505572734652, 2.5165947299310134, 2.4160217622690503, 2.2805528204062417, 2.118993220301145, 1.9460351195674463, 1.7862411461060212], "Full track array"=w33, "Multiline grouping, samples"=w24, "Samples full merge, every N"=w23, "error in (no error)"=w1) -> ("Speed-coded overlay refnum out"=→"Image Display":T1, "error out"=w31:errorcluster)  [unwired: 8 in]
  n9 = call "GEN_Time-coded_overlay.vi"("Time-coded overlay refnum in"=w25, "Full track array"=w33, "Multiline grouping, samples"=w24, "Samples full merge, every N"=w23, "error in (no error)"=w16) -> ("Time-coded overlay refnum out"=→"Image Display 2":T1, "error out"=w30:errorcluster)  [unwired: 9 in]
  n10 = Merge Errors(w31, w30) -> (→"error out":errorcluster)
  "Color" <- w5
